vi "Graphics.Read Image File and Auto Scale for 2D Picture.vi"(8 "error in (no error)":errorcluster, 10 "2D Pict Ref":refnum<vi>, 11 "File":path) -> (0 "error out":errorcluster, 1 "image data":T1, 2 "Zoom Factor":dbl, 3 "2D Pict":picture)   [LabVIEW 2024, in "EQMF.lvlib" / "Graphic Utils.lvlib"]
uses:
  Graphic Utils.lvlib
  <vilib>/picture/picture.llb/imagedata.ctl
  <vilib>/Utility/miscctls.llb/LVPointTypeDef.ctl
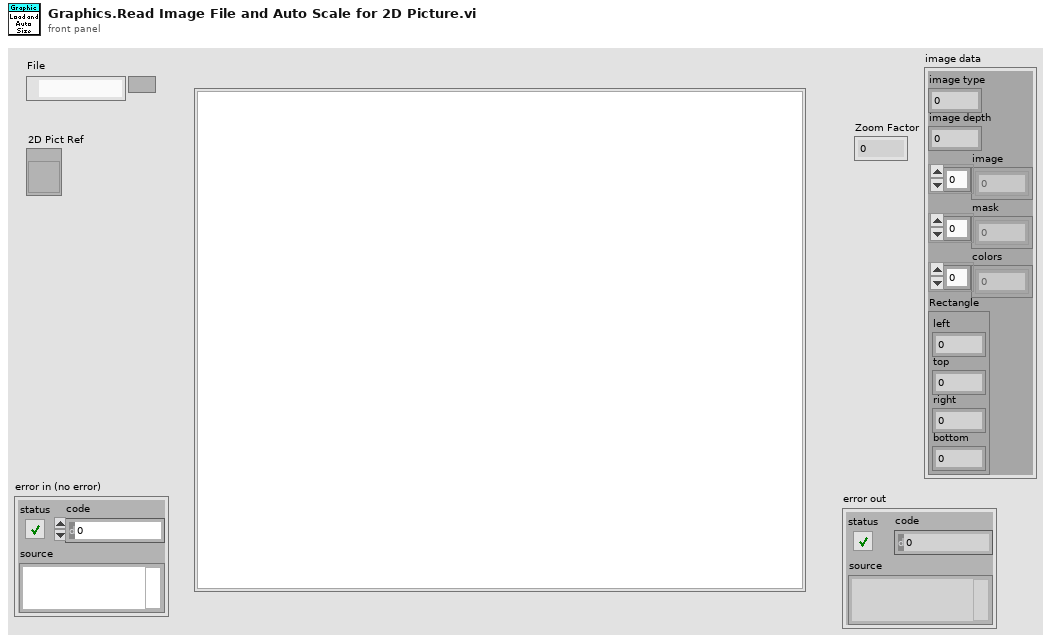
[diagram p1: front panel]
types:
  T1 = typedef "imagedata.ctl" = cluster{"image type":i32, "image depth":i32, "image":u8[], "mask":u8[], "colors":u32[], "Rectangle":cluster{"left":i16, "top":i16, "right":i16, "bottom":i16}}
  T2 = typedef "LVPointTypeDef.ctl" = cluster{"Horizontal":i16, "Vertical":i16}
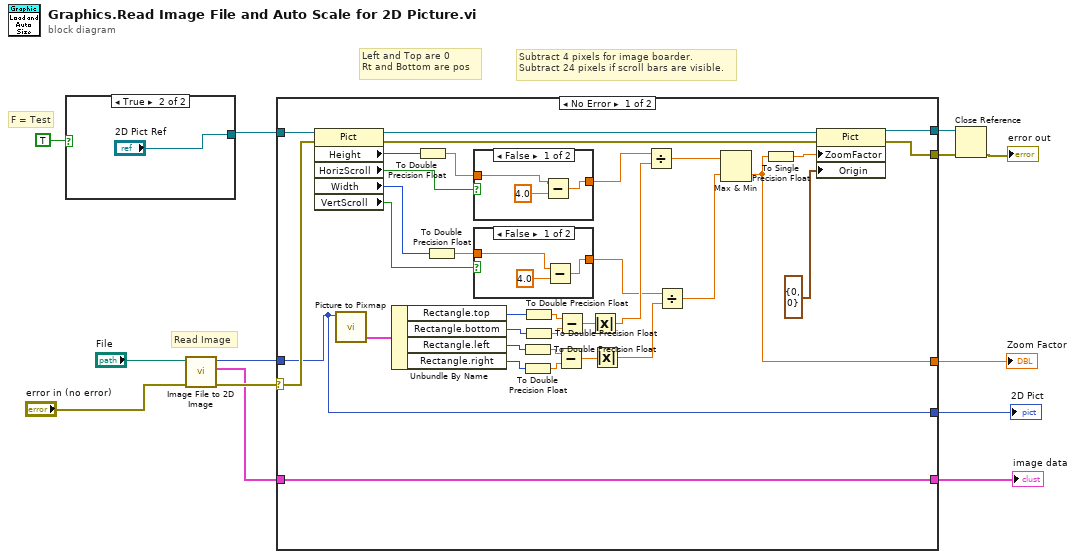
[diagram p0: block diagram]
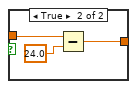
[diagram p2: hidden frame]
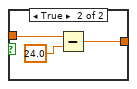
[diagram p3: hidden frame]
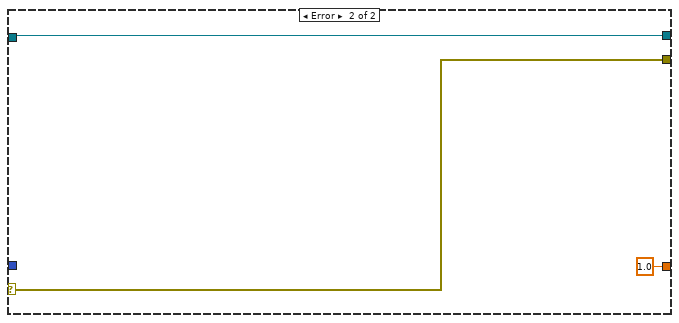
[diagram p4: hidden frame]
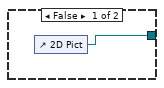
[diagram p5: hidden frame]
diagram:
  # "Subtract 4 pixels for image boarder.\nSubtract 24 pixels if scroll bars are visible."
  # "F = Test"
  # "Left and Top are 0\nRt and Bottom are pos"
  # "Read Image"
  n1 = case shown="True" TRUE {
    tunnel: [w14 "2D Pict Ref"] -> w11
    frame False {
      n2 = control-ref of="2D Pict"() -> (w14:refnum<vi>)
    }
    frame True {
    }
  }
  n3 = call "Image File to 2D Image.vi"("error in"="error in (no error)", "Path"="File") -> ("error out"=w7:errorcluster, "image data"=w3:T1, "2D Picture"=w8:picture)  [unwired: 7 in]
  n4 = case shown="No Error" w7 {
    selector: w7 -> [w39 w63]
    tunnel: w11 -> [w48 w64]
    tunnel: [w41 1.0] -> w10
    tunnel: w8 -> [w16 _]
    tunnel: [w38 w64] -> w6
    tunnel: [w37 w63] -> w5
    tunnel: w3 -> [w17 _]
    tunnel: [w17 _] -> w2
    tunnel: [w16 _] -> w1
    frame No Error {
      n5 = property on="Property Node" class="Pict"(reference=w48, error in=w39) -> (reference out=w43:refnum<vi>, error out=w40:errorcluster, "Height"=w47:u32, "HorizScroll"=w23:bool, "Width"=w46:u32, "VertScroll"=w19:bool)
      n6 = call <vilib>:"Picture to Pixmap.vi"("picture"=w16) -> ("image data"=w49:T1)  [unwired: 9 in, 1 out]
      n7 = Unbundle By Name(w49) -> ("Rectangle.top"=w30:i16, "Rectangle.bottom"=w31:i16, "Rectangle.left"=w32:i16, "Rectangle.right"=w29:i16)
      n8 = To Double Precision Float(number=w47) -> (double precision float=w22:dbl)
      n9 = To Double Precision Float(number=w46) -> (double precision float=w20:dbl)
      n10 = case shown="False" w23 {
        tunnel: w22 -> [w58 w60]
        tunnel: [w56 w59] -> w21
        frame False {
          n11 = Subtract(x=w58, y=4.0) -> (x-y=w56:dbl)
        }
        frame True {
          n12 = Subtract(x=w60, y=24.0) -> (x-y=w59:dbl)
        }
      }
      n13 = case shown="False" w19 {
        tunnel: w20 -> [w51 w54]
        tunnel: [w50 w53] -> w18
        frame False {
          n14 = Subtract(x=w51, y=4.0) -> (x-y=w50:dbl)
        }
        frame True {
          n15 = Subtract(x=w54, y=24.0) -> (x-y=w53:dbl)
        }
      }
      n16 = To Double Precision Float(number=w32) -> (double precision float=w35:dbl)
      n17 = To Double Precision Float(number=w29) -> (double precision float=w36:dbl)
      n18 = To Double Precision Float(number=w30) -> (double precision float=w34:dbl)
      n19 = To Double Precision Float(number=w31) -> (double precision float=w33:dbl)
      n20 = Subtract(x=w35, y=w36) -> (x-y=w27:dbl)
      n21 = Subtract(x=w34, y=w33) -> (x-y=w28:dbl)
      n22 = Absolute Value(x=w28) -> (abs(x)=w26:dbl)
      n23 = Absolute Value(x=w27) -> (abs(x)=w25:dbl)
      n24 = Divide(x=w21, y=w26) -> (x/y=w45:dbl)
      n25 = Divide(x=w18, y=w25) -> (x/y=w44:dbl)
      n26 = Max & Min(x=w45, y=w44) -> (min(x,y)=w41:dbl)  [unwired: 1 out]
      n27 = To Single Precision Float(number=w41) -> (single precision float=w42:sgl)
      n28 = property on="Property Node" class="Pict"(reference=w43, error in=w40, "ZoomFactor"=w42, "Origin"=T2 {"Horizontal"=0, "Vertical"=0}) -> (reference out=w38:refnum<vi>, error out=w37:errorcluster)
    }
    frame Error {
    }
  }
  "Zoom Factor" <- w10
  "2D Pict" <- w1
  "image data" <- w2
  n29 = Close Reference(reference=w6, error in (no error)=w5) -> (error out=→"error out":errorcluster)
